vi "Giradinha3 (SubVI).vi"(9 "Raio":dbl=300.0, 10 "Robot in":refnum<class "Robot.lvclass">=refnum, 11 "Game in":refnum<class "Game.lvclass">=refnum) -> (2 "Estado":string="Indo ate a circunferencia", 3 "Robot out":refnum<class "Robot.lvclass">)   [LabVIEW 2021]
uses:
  Game_class/Game.lvclass
  Robot_class/Robot.lvclass
  C:/Users/IME/Desktop/Horie - VSS - SSL/SSL_AI/Object_class/Object.lvclass
  Ally_class/Ally.lvclass
  Ball_class/Ball.lvclass
  Referee_class/Referee.lvclass
  Field_class/Field.lvclass
  Enemy_class/Enemy.lvclass
  Events_class/Events.lvclass
  Utilities_class/Utilities.lvclass
  Parameters_class/Parameters.lvclass
  Playbook_class/Playbook.lvclass
  Play_class/Play.lvclass
  TestPlay_class/TestPlay.lvclass
  EnemyPossessionAtEnemyFieldPlay_class/EnemyPossessionAtEnemyFieldPlay.lvclass
  EnemyPossessionAtOurFieldPlay_class/EnemyPossessionAtOurFieldPlay.lvclass
  NormalGamePlay_class/NormalGamePlay.lvclass
  IndirectEnemyPlay_class/IndirectEnemyPlay.lvclass
  PrepareKickoffAllyPlay_class/PrepareKickoffAllyPlay.lvclass
  PrepareKickoffEnemyPlay_class/PrepareKickoffEnemyPlay.lvclass
  KickPenaltyAllyPlay_class/KickPenaltyAllyPlay.lvclass
  PreparePenaltyAllyPlay_class/PreparePenaltyAllyPlay.lvclass
  DirectEnemyPlay_class/DirectEnemyPlay.lvclass
  PreparePenaltyEnemyPlay_class/PreparePenaltyEnemyPlay.lvclass
  BallOutOfFieldPlay_class/BallOutOfFieldPlay.lvclass
  StopOffensivePlay_class/StopOffensivePlay.lvclass
  PassPlay_class/PassPlay.lvclass
  DirectKickPlay_class/DirectKickPlay.lvclass
  HaltPlay_class/HaltPlay.lvclass
  PreparePassPlay_class/PreparePassPlay.lvclass
  PassToStriker_class/PassToStriker.lvclass
  PassTo2ndStriker_class/PassTo2ndStriker.lvclass
  SimplePass_class/SimplePass.lvclass
  PrepareRollToPassPlay_class/PrepareRollToPassPlay.lvclass
  PrepareDoublePassPlay_class/PrepareDoublePassPlay.lvclass
  TableWith2ndStrikerPlay_class/TableWith2ndStrikerPlay.lvclass
  TableWithStrikerPlay_class/TableWithStrikerPlay.lvclass
  PrepareTriplePassPlay_class/PrepareTriplePassPlay.lvclass
  ABCPassPlay_class/ABCPassPlay.lvclass
  PreparePassInGame1_class/PreparePassInGame1.lvclass
  ACBPassPlay_class/ACBPassPlay.lvclass
  PrepareKeeperPassPlay_class/PrepareKeeperPassPlay.lvclass
  KeeperPassToStrikerPlay_class/KeeperPassToStrikerPlay.lvclass
  5RobotsNormalGamePlay_class/5RobotsNormalGamePlay.lvclass
  Rolebook_class/Rolebook.lvclass
  5RobotsRole_class/5RobotsRole.lvclass
  Tacticbook_class/Tacticbook.lvclass
  ShootRole_class/ShootRole.lvclass
  5RobotsPassGamePlay_class/5RobotsPassGamePlay.lvclass
  PassBestRobotRole_class/PassBestRobotRole.lvclass
  PassBestReceiverRole_class/PassBestReceiverRole.lvclass
  5RobotsKeeperGame_class/5RobotsKeeperGame.lvclass
  5PreparePassGamePlay_class/5PreparePassGamePlay.lvclass
  NormalDefensivePlay_class/NormalDefensivePlay.lvclass
  NormalDefensiveWithDuelistPlay_class/NormalDefensiveWithDuelistPlay.lvclass
  KeeperPlay_class/KeeperPlay.lvclass
  KeeperRole_class/KeeperRole.lvclass
  TimeoutPlay_class/TimeoutPlay.lvclass
  ZigZagPlay_class/ZigZagPlay.lvclass
  GoToPlay_class/GoToPlay.lvclass
  BallPlacementPlay_class/BallPlacementPlay.lvclass
  BallPlacementAllyPlay_class/BallPlacementAllyPlay.lvclass
  SimpleBallPlacementAllyPlay_class/SimpleBallPlacementAllyPlay.lvclass
  RobotFeedback/RobotFeedback.lvclass
  Control 3.ctl
  Game_class/Game.lvclass/Game.ctl
  Object_class/Object.lvclass/Object.ctl
  Robot_class/Robot.lvclass/Robot.ctl
  <vilib>/Analysis/baseanly.llb/Unit Vector (DBL).vi
  <vilib>/Analysis/coordinate.llb/2D Cartesian Coordinate Rotation (Scalar).vi
  Object_class/Read position(x,y).vi
  Game_class/Read BallRef.vi
  Game_class/Read FieldRef.vi
  Object_class/Read x.vi
  Object_class/Read y.vi
  Robot_class/Write dest_orientation.vi
  Robot_class/Write dest_x.vi
  Robot_class/Write dest_y.vi
  Robot_class/Write kick_x.vi
  <vilib>/Analysis/NI_AALBase.lvlib
  <vilib>/Analysis/NI_AALPro.lvlib
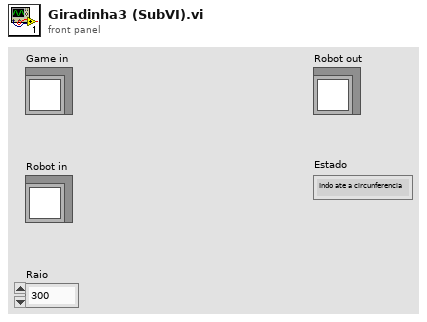
[diagram p1: front panel]
types:
  T1 = typedef "Control 3.ctl" = enum16{"Indo ate a circunferencia", "Girando", "Chutando"}
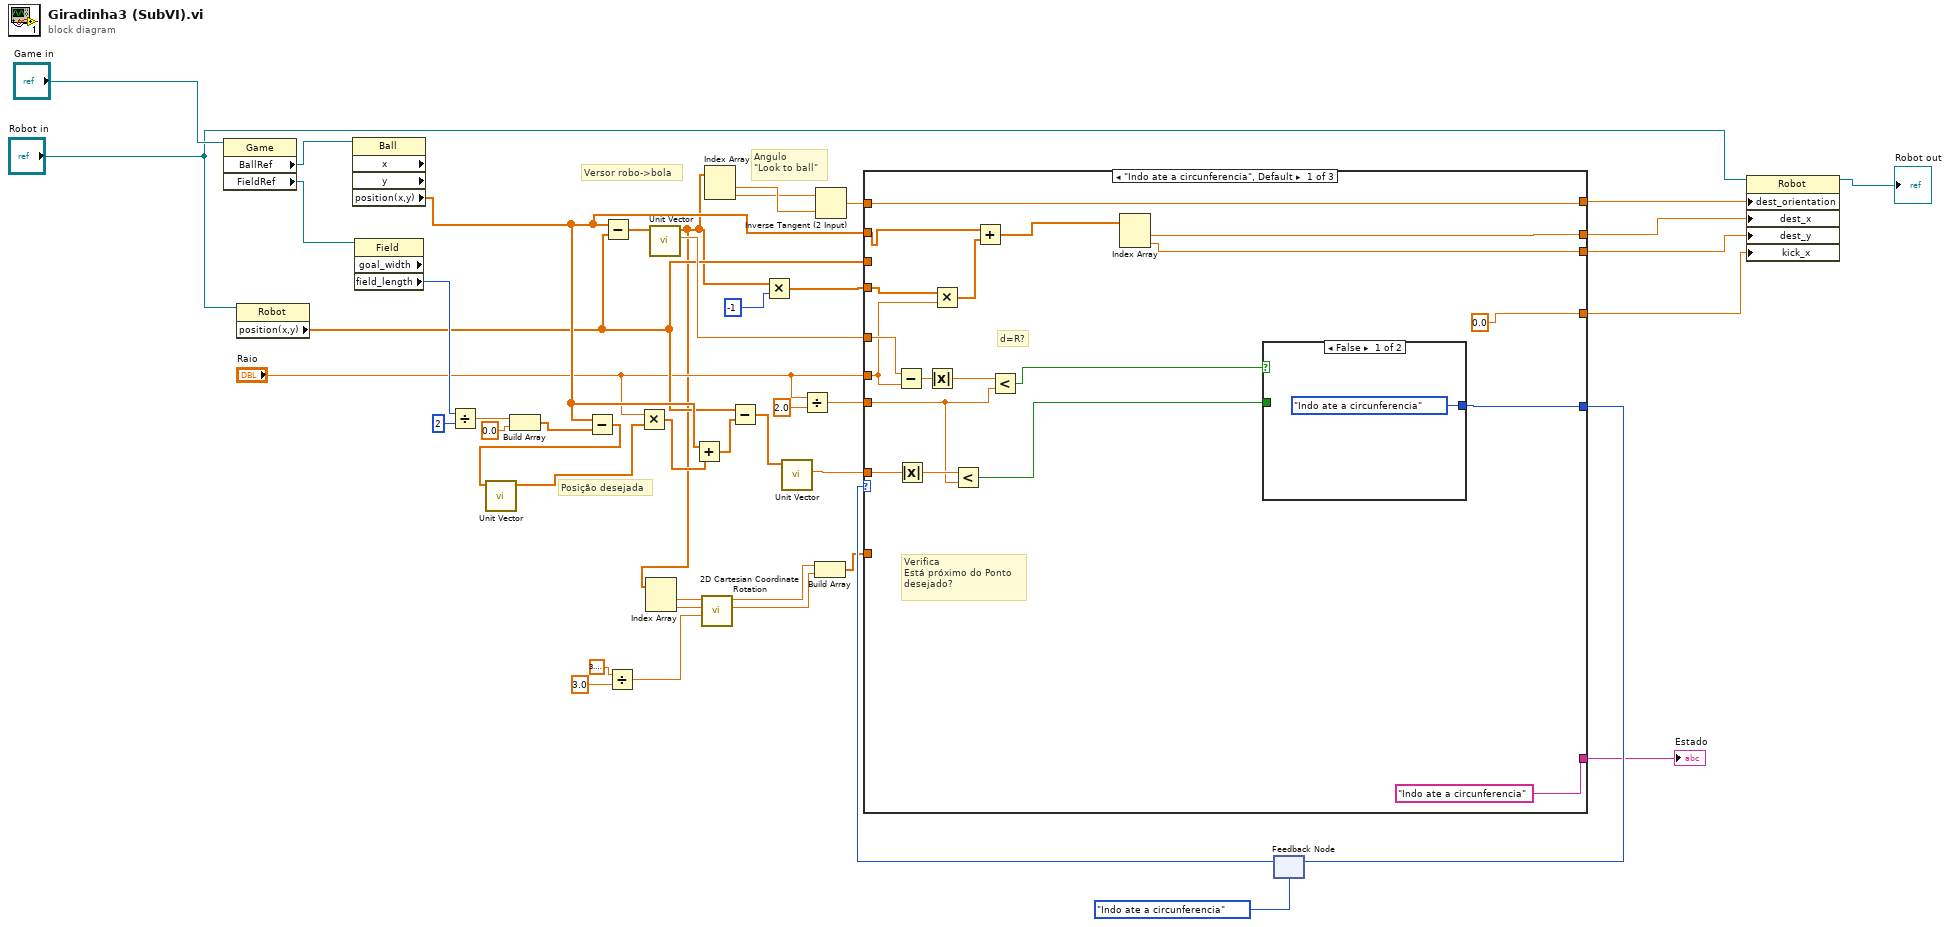
[diagram p0: block diagram]
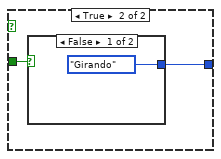
[diagram p2: hidden frame]
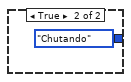
[diagram p3: hidden frame]
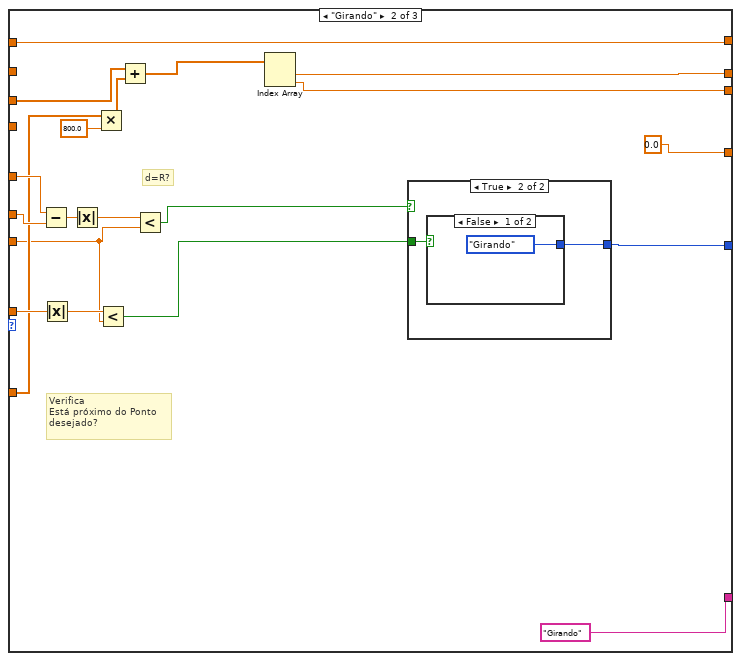
[diagram p4: hidden frame]
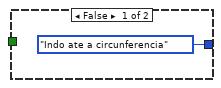
[diagram p5: hidden frame]
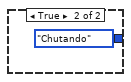
[diagram p6: hidden frame]
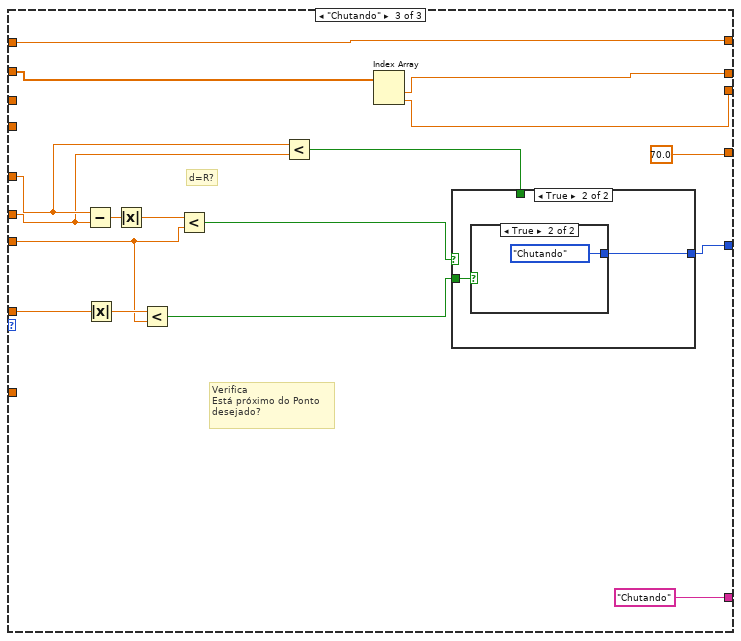
[diagram p7: hidden frame]
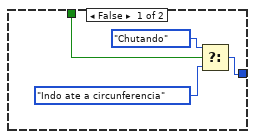
[diagram p8: hidden frame]
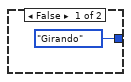
[diagram p9: hidden frame]
diagram:
  # "Posição desejada"
  # "Versor robo->bola"
  # "Angulo\n\"Look to ball\""
  n1 = property class="Game"(reference="Game in") -> ("BallRef"=w44:refnum<class "Ball.lvclass">, "FieldRef"=w43:refnum<class "Field.lvclass">)  [unwired: 1 in, 2 out]
  n2 = property class="Robot"(reference="Robot in") -> ("position(x,y)"=w13:dbl[])  [unwired: 1 in, 2 out]
  n3 = property class="Ball" props=["x", "y", "position(x,y)"](reference=w44) -> ("position(x,y)"=w15:dbl[])  [unwired: 1 in, 4 out]
  n4 = property class="Field" props=["goal_width", "field_length"](reference=w43) -> ("field_length"=w34:i32)  [unwired: 1 in, 3 out]
  n5 = Divide(x=w34, y=2) -> (x/y=w32:dbl)
  n6 = Build Array(w32, 0.0 ("element")) -> (w30:dbl[])
  n7 = Subtract(x=w15, y=w30) -> (x-y=w19:dbl[])
  n8 = call-poly <vilib>:"Unit Vector.vi"("Input Vector"=w19) -> ("Unit Vector"=w18:dbl[])  [unwired: 8 in, 2 out]
  n9 = Subtract(x=w15, y=w13) -> (x-y=w41:dbl[])
  n10 = Divide(x=3.141592653589793, y=3.0) -> (x/y=w4:dbl)
  n11 = Multiply(x="Raio", y=w18) -> (x*y=w17:dbl[])
  n12 = call-poly <vilib>:"Unit Vector.vi"("Input Vector"=w41) -> ("norm"=w35:dbl, "Unit Vector"=w9:dbl[])  [unwired: 8 in, 1 out]
  n13 = Index Array(array=w9) -> (element #1=w8:dbl, element #2=w7:dbl)  [unwired: 2 in]
  n14 = Add(x=w15, y=w17) -> (x+y=w16:dbl[])
  n15 = call-poly <vilib>:"2D Cartesian Coordinate Rotation.vi"("theta"=w4, "y"=w7, "x"=w8) -> ("y out"=w2:dbl, "x out"=w3:dbl)  [unwired: 6 in, 1 out]
  n16 = Index Array(array=w9) -> (element #1=w40:dbl, element #2=w39:dbl)  [unwired: 2 in]
  n17 = Subtract(x=w13, y=w16) -> (x-y=w22:dbl[])
  n18 = Multiply(x=w9, y=-1) -> (x*y=w29:dbl[])
  n19 = call-poly <vilib>:"Unit Vector.vi"("Input Vector"=w22) -> ("norm"=w21:dbl)  [unwired: 8 in, 2 out]
  n20 = Divide(x="Raio", y=2.0) -> (x/y=w10:dbl)
  n21 = Build Array(w3, w2) -> (w14:dbl[])
  n22 = Inverse Tangent (2 Input)(1:w40, 2:w39) -> (0:w38:dbl)
  n23 = feedback #1(Control_3."Indo ate a circunferencia") -> (w42:T1)
  n24 = case shown="\"Indo ate a circunferencia\", Default" w42 {
    tunnel: [w62 w88 w103] -> w24
    tunnel: w38 -> [w64 w89 w111]
    tunnel: [w64 w89 w111] -> w36
    tunnel: w29 -> [w63 _ _]
    tunnel: "Raio" -> [w55 w81 w98]
    tunnel: w35 -> [w58 w84 w99]
    tunnel: w14 -> [_ w74 _]
    tunnel: [w61 w87 w101] -> w27
    tunnel: [w60 w86 w100] -> w26
    tunnel: ["Indo ate a circunferencia" "Girando" "Chutando"] -> w23
    tunnel: w21 -> [w52 w78 w104]
    tunnel: w15 -> [w50 _ w102]
    tunnel: w13 -> [_ w75 _]
    tunnel: w10 -> [w47 w71 w96]
    tunnel: [0.0 0.0 70.0] -> w1
    frame "Indo ate a circunferencia", Default {
      # "Verifica\nEstá próximo do Ponto\ndesejado?"
      # "d=R?"
      n25 = Subtract(x=w58, y=w55) -> (x-y=w57:dbl)
      n26 = Absolute Value(x=w52) -> (abs(x)=w51:dbl)
      n27 = Absolute Value(x=w57) -> (abs(x)=w56:dbl)
      n28 = Multiply(x=w63, y=w55) -> (x*y=w49:dbl[])
      n29 = Less?(x=w51, y=w47) -> (x < y?=w53:bool)
      n30 = Add(x=w50, y=w49) -> (x+y=w48:dbl[])
      n31 = Less?(x=w56, y=w47) -> (x < y?=w54:bool)
      n32 = Index Array(array=w48) -> (element #1=w61:dbl, element #2=w60:dbl)  [unwired: 2 in]
      n33 = case shown="False" w54 {
        tunnel: [Control_3."Indo ate a circunferencia" w67] -> w62
        tunnel: w53 -> [_ w66]
        frame False {
        }
        frame True {
          n34 = case shown="False" w66 {
            tunnel: [Control_3."Girando" Control_3."Chutando"] -> w67
            frame False {
            }
            frame True {
            }
          }
        }
      }
    }
    frame "Girando" {
      # "Verifica\nEstá próximo do Ponto\ndesejado?"
      # "d=R?"
      n35 = Subtract(x=w84, y=w81) -> (x-y=w83:dbl)
      n36 = Absolute Value(x=w78) -> (abs(x)=w77:dbl)
      n37 = Absolute Value(x=w83) -> (abs(x)=w82:dbl)
      n38 = Multiply(x=w74, y=800.0) -> (x*y=w73:dbl[])
      n39 = Less?(x=w77, y=w71) -> (x < y?=w79:bool)
      n40 = Add(x=w75, y=w73) -> (x+y=w76:dbl[])
      n41 = Less?(x=w82, y=w71) -> (x < y?=w80:bool)
      n42 = Index Array(array=w76) -> (element #1=w87:dbl, element #2=w86:dbl)  [unwired: 2 in]
      n43 = case shown="True" w80 {
        tunnel: [Control_3."Indo ate a circunferencia" w92] -> w88
        tunnel: w79 -> [_ w91]
        frame False {
        }
        frame True {
          n44 = case shown="False" w91 {
            tunnel: [Control_3."Girando" Control_3."Chutando"] -> w92
            frame False {
            }
            frame True {
            }
          }
        }
      }
    }
    frame "Chutando" {
      # "Verifica\nEstá próximo do Ponto\ndesejado?"
      # "d=R?"
      n45 = Subtract(x=w99, y=w98) -> (x-y=w109:dbl)
      n46 = Absolute Value(x=w104) -> (abs(x)=w105:dbl)
      n47 = Absolute Value(x=w109) -> (abs(x)=w108:dbl)
      n48 = Less?(x=w105, y=w96) -> (x < y?=w106:bool)
      n49 = Less?(x=w108, y=w96) -> (x < y?=w107:bool)
      n50 = Less?(x=w99, y=w98) -> (x < y?=w97:bool)
      n51 = Index Array(array=w102) -> (element #1=w101:dbl, element #2=w100:dbl)  [unwired: 2 in]
      n52 = case shown="True" w107 {
        tunnel: [w113 w117] -> w103
        tunnel: w106 -> [_ w116]
        tunnel: w97 -> [w112 _]
        frame False {
          n53 = Select(t=Control_3."Chutando", s=w112, f=Control_3."Indo ate a circunferencia") -> (s? t:f=w113:T1)
        }
        frame True {
          n54 = case shown="True" w116 {
            tunnel: [Control_3."Girando" Control_3."Chutando"] -> w117
            frame False {
            }
            frame True {
            }
          }
        }
      }
    }
  }
  "Estado" <- w23
  n55 = feedback-in #1(w24) -> ()
  n56 = property class="Robot"(reference="Robot in", "dest_orientation"=w36, "dest_x"=w27, "dest_y"=w26, "kick_x"=w1) -> (reference out=→"Robot out":refnum<class "Robot.lvclass">)  [unwired: 1 in, 1 out]
